vi "filter_logic_delays.vi"(9 "Filter Specific Constants":T2, 10 "Variables Cluster":T4, 11 "controls cluster":T1={"High Charge Limit"=0, "Low Charge Limit"=0, "Time Out Limit"=0, "High Velocity Count"=0, "Low Velocity Count"=0, "Sampling Rate"=26666666.59375, "High Mass Limit"=0, "Low Mass Limit"=0}) -> (3 "Output Cluster":T3)   [LabVIEW 2013]
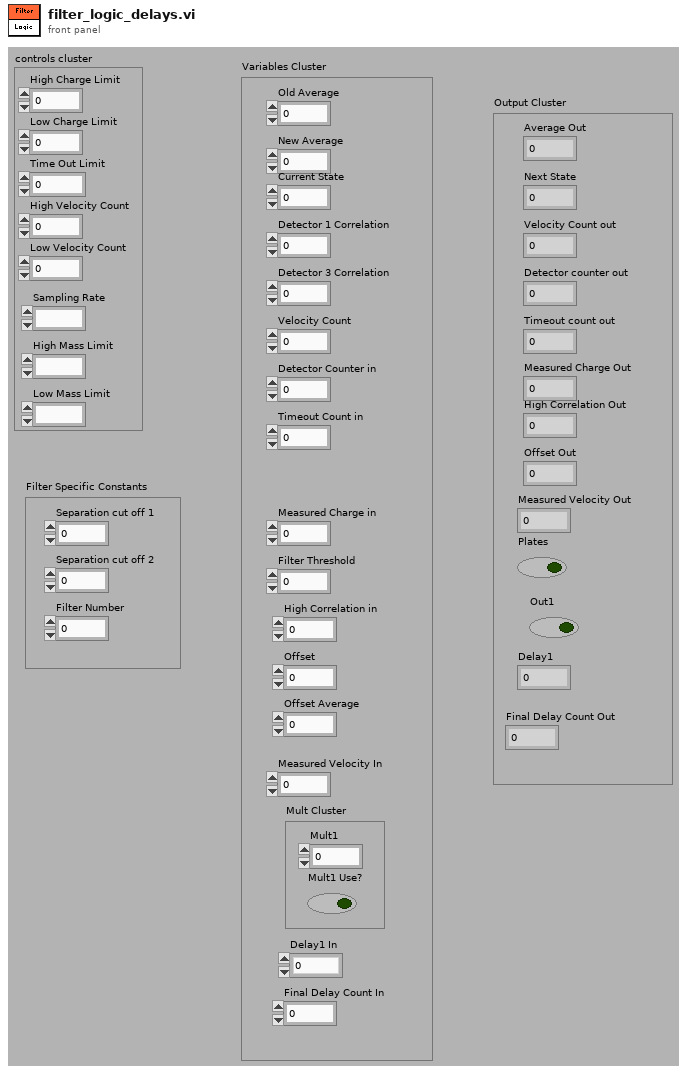
[diagram p1: front panel]
types:
  T1 = cluster{"High Charge Limit":i16, "Low Charge Limit":i16, "Time Out Limit":i32, "High Velocity Count":i32, "Low Velocity Count":i32, "Sampling Rate":fxp<+,30,25>, "High Mass Limit":i64, "Low Mass Limit":i64}
  T2 = cluster{"Separation cut off 1":i32, "Filter Number":i32, "Separation cut off 2":i32}
  T3 = cluster{"Average Out":i32, "Next State":u8, "Velocity Count out":i32, "Detector counter out":i32, "Timeout count out":u32, "Measured Charge Out":i32, "High Correlation Out":i32, "Plates":bool, "Offset Out":i32, "Measured Velocity Out":i32, "Final Delay Count Out":u16, "Out1":bool, "Delay1":i32}
  T4 = cluster{"Old Average":i32, "New Average":i32, "Current State":u8, "Detector 1 Correlation":i32, "Detector 3 Correlation":i32, "Velocity Count":i32, "Detector Counter in":i32, "Timeout Count in":i32, "Measured Charge in":i32, "Filter Threshold":i32, "High Correlation in":i32, "Offset":i32, "Offset Average":i32, "Measured Velocity In":i32, "Mult Cluster":cluster{"Mult1":fxp<+,16,7>, "Mult1 Use?":bool}, "Final Delay Count In":u16, "Delay1 In":i32}
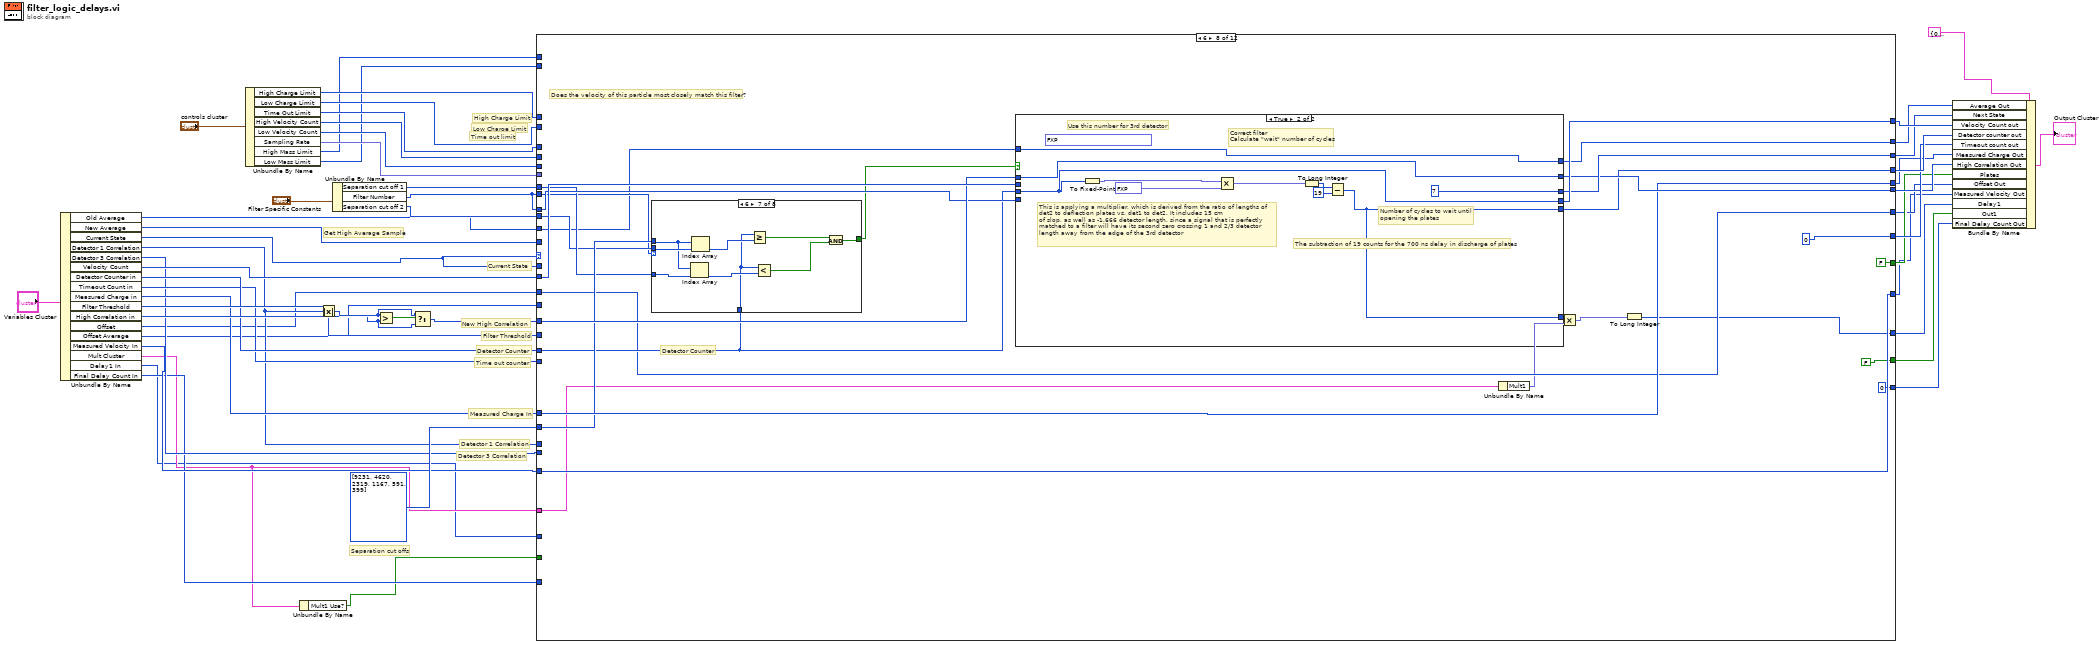
[diagram p0: block diagram]
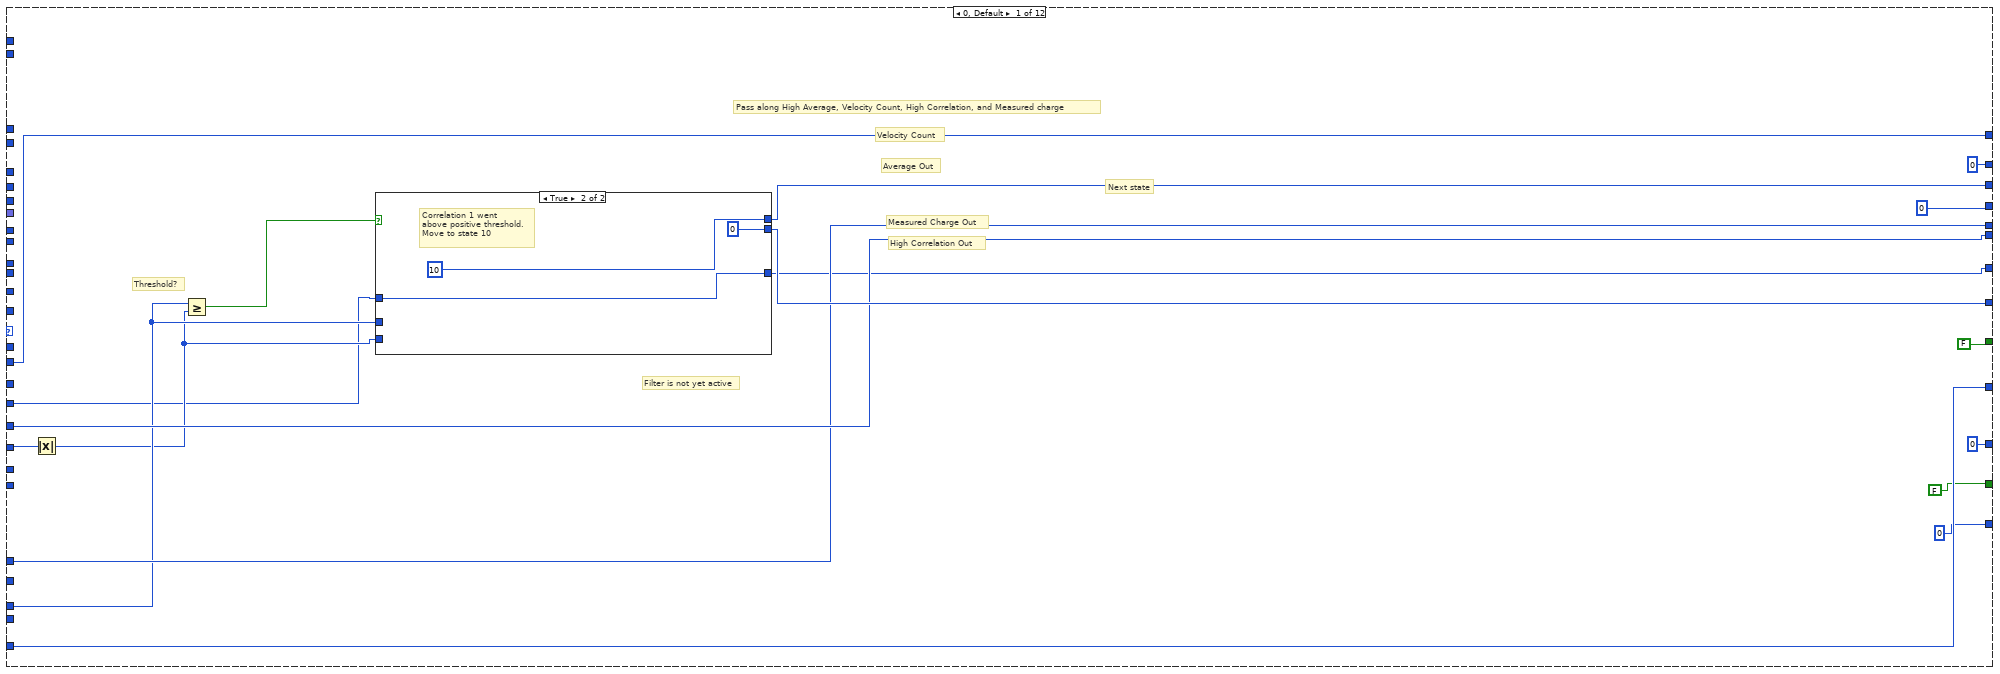
[diagram p2: hidden frame]
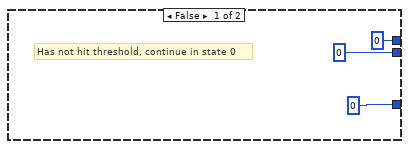
[diagram p3: hidden frame]
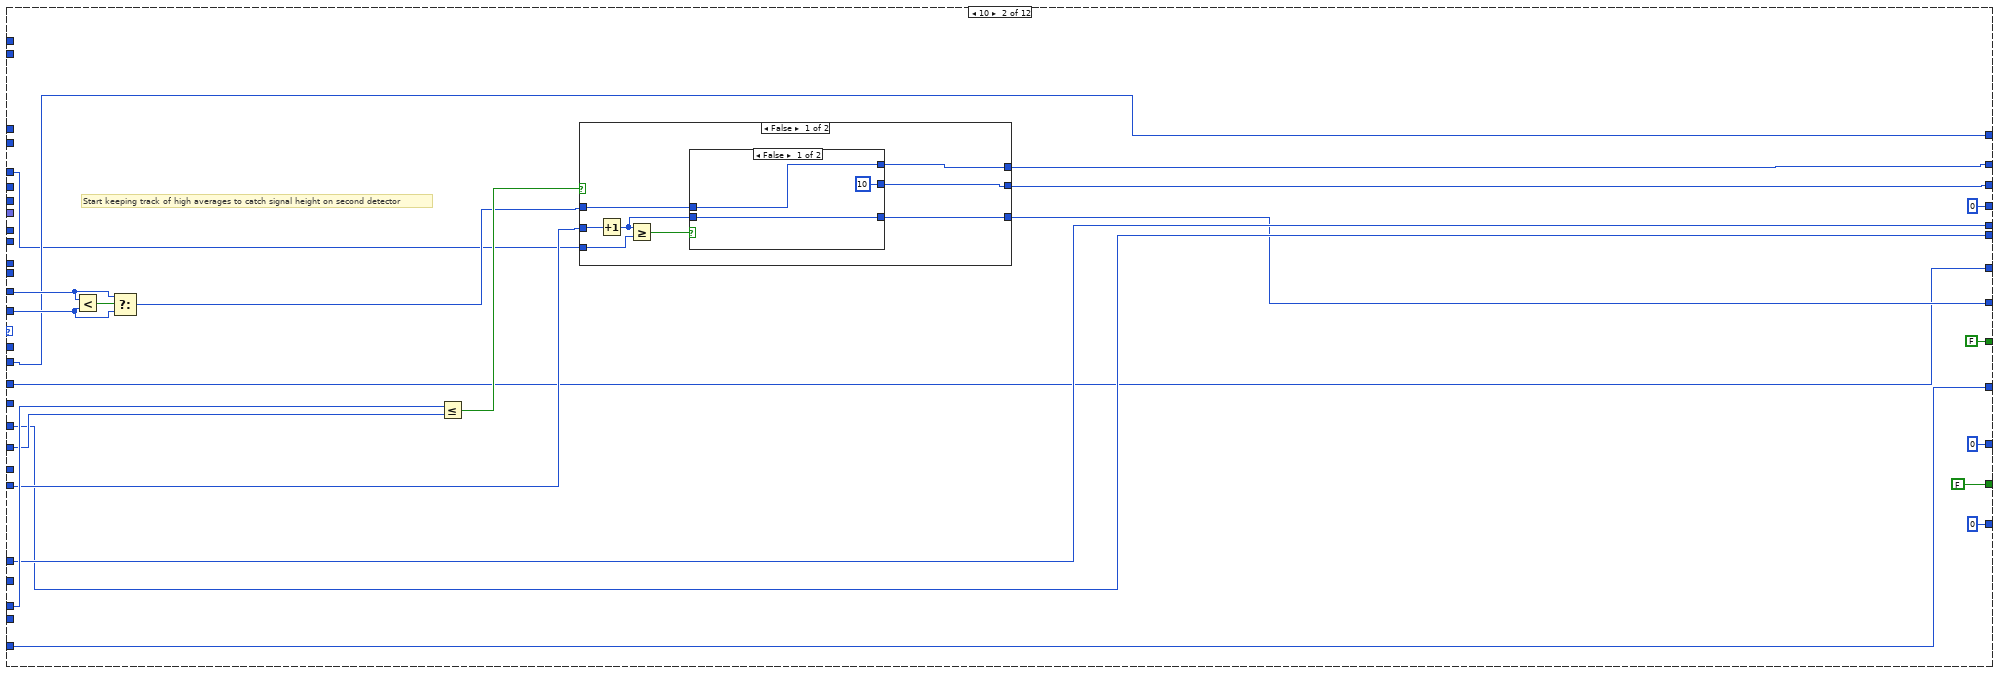
[diagram p4: hidden frame]
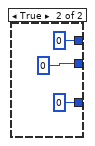
[diagram p5: hidden frame]
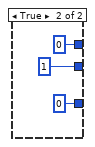
[diagram p6: hidden frame]
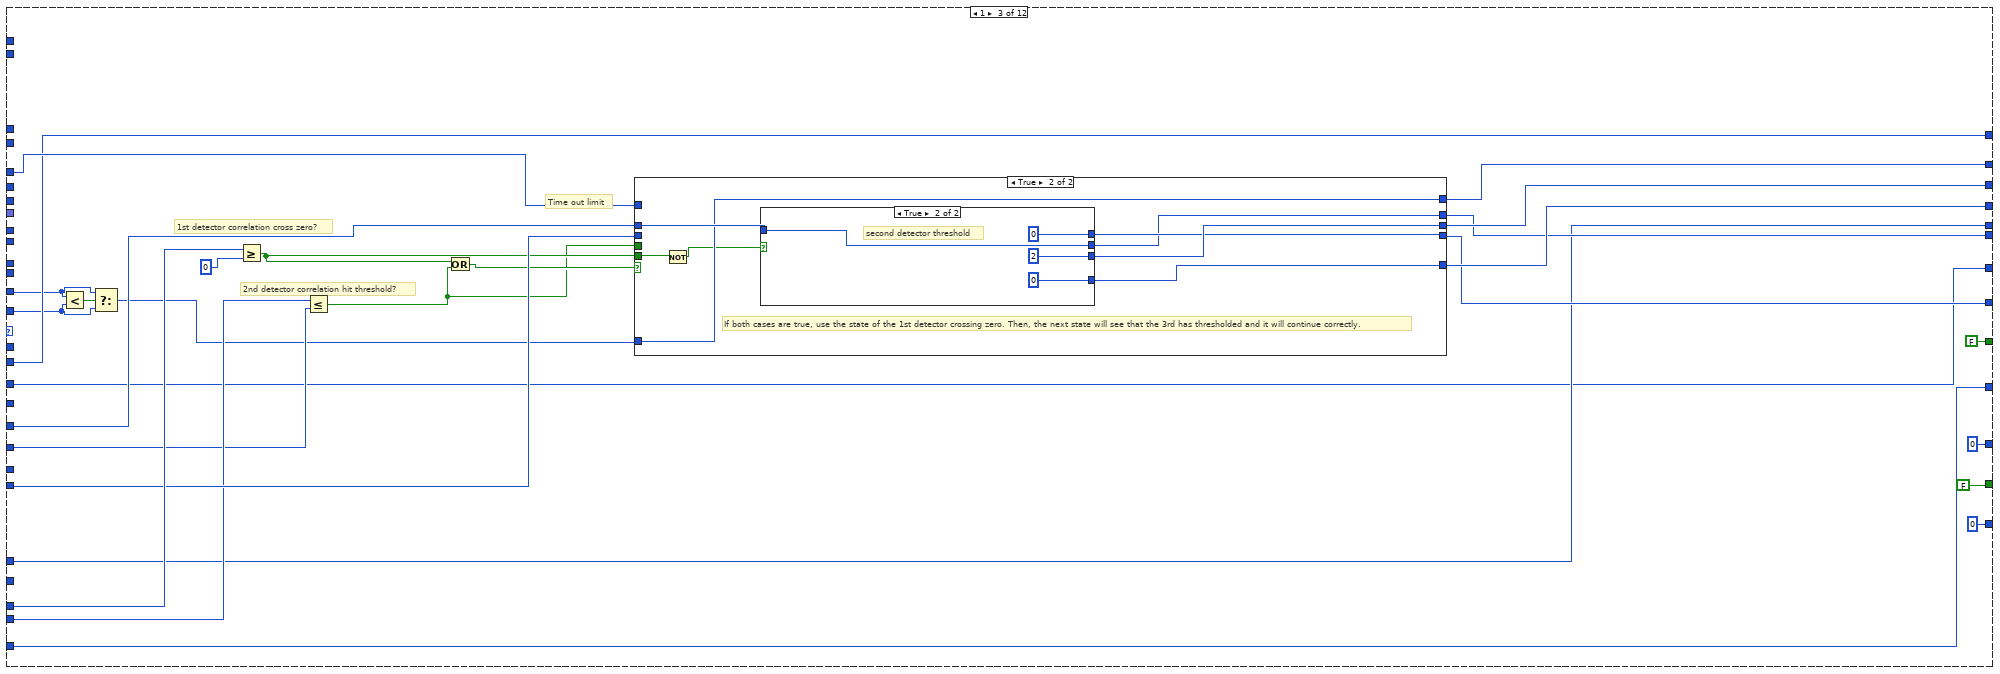
[diagram p7: hidden frame]
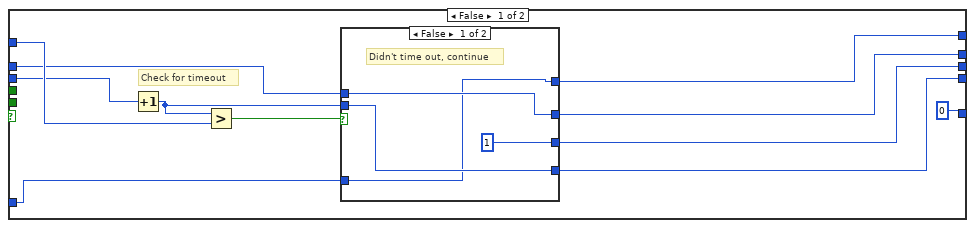
[diagram p8: hidden frame]
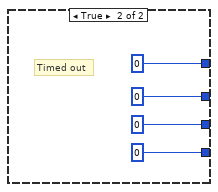
[diagram p9: hidden frame]
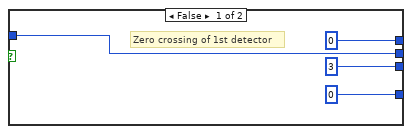
[diagram p10: hidden frame]
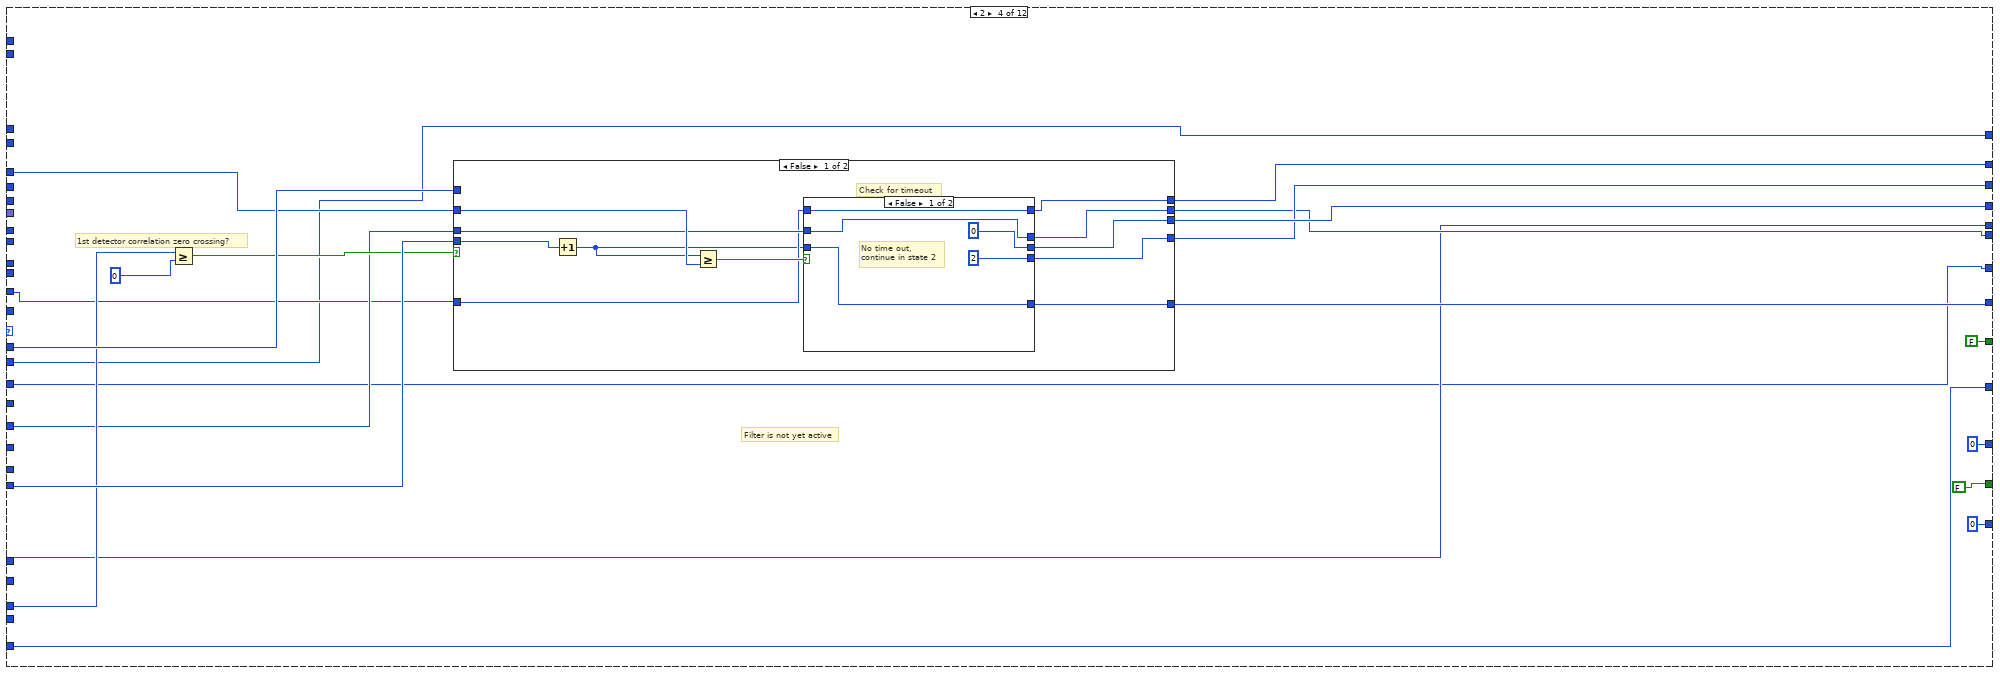
[diagram p11: hidden frame]
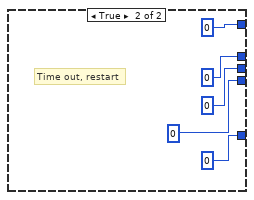
[diagram p12: hidden frame]
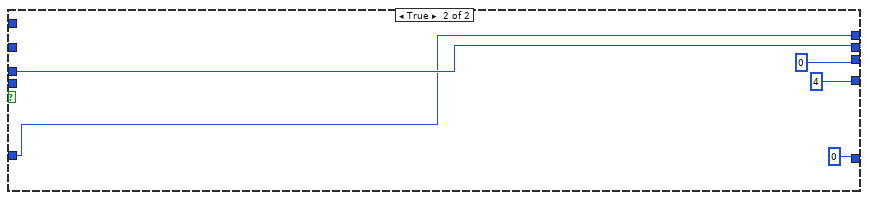
[diagram p13: hidden frame]
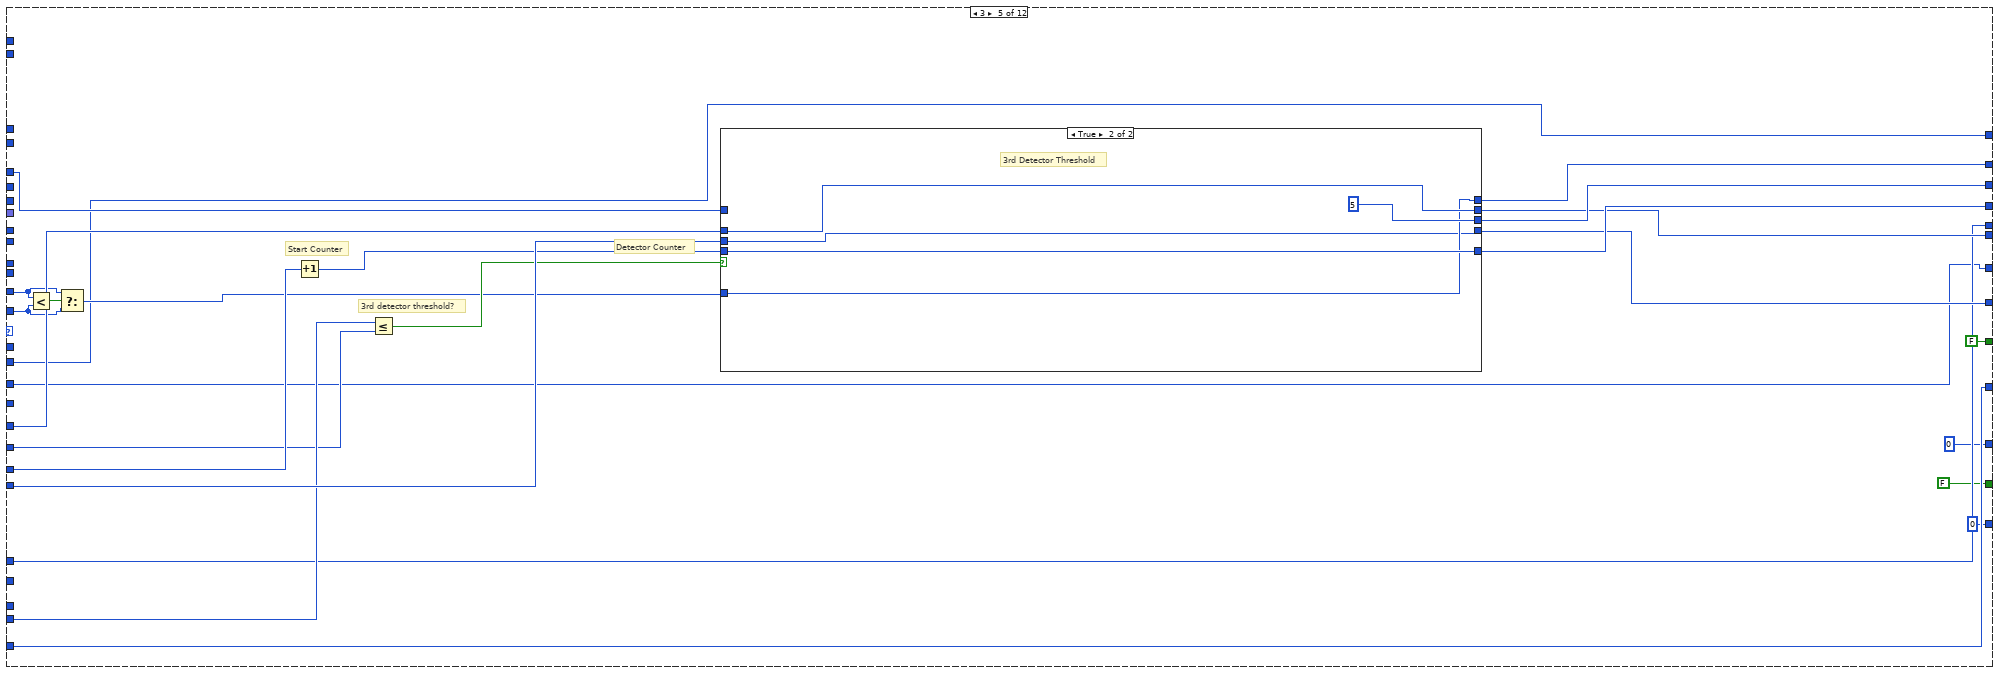
[diagram p14: hidden frame]
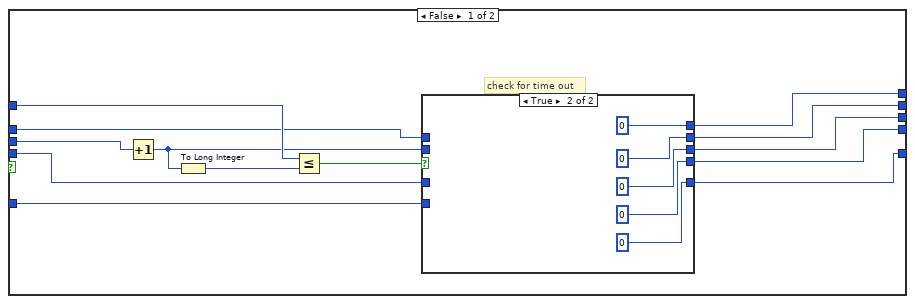
[diagram p15: hidden frame]
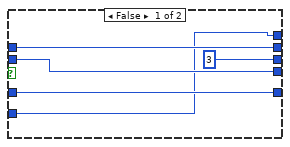
[diagram p16: hidden frame]
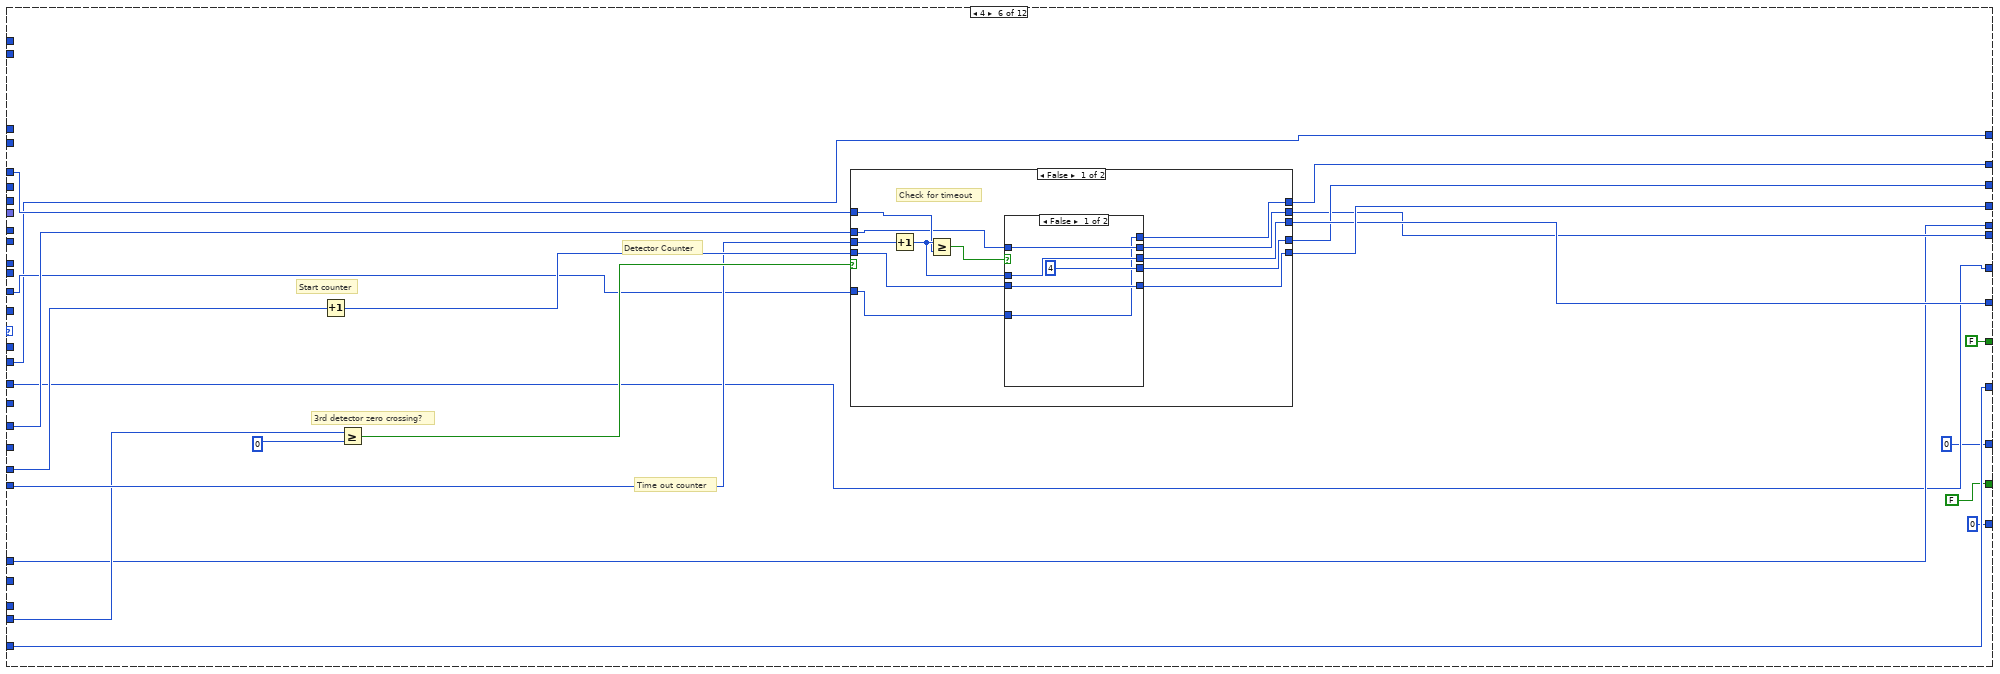
[diagram p17: hidden frame]
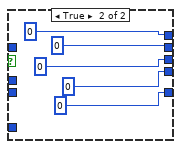
[diagram p18: hidden frame]
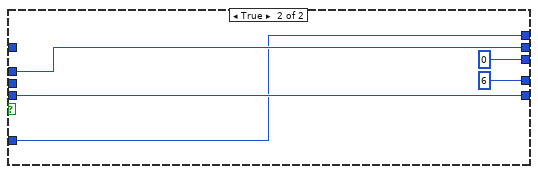
[diagram p19: hidden frame]
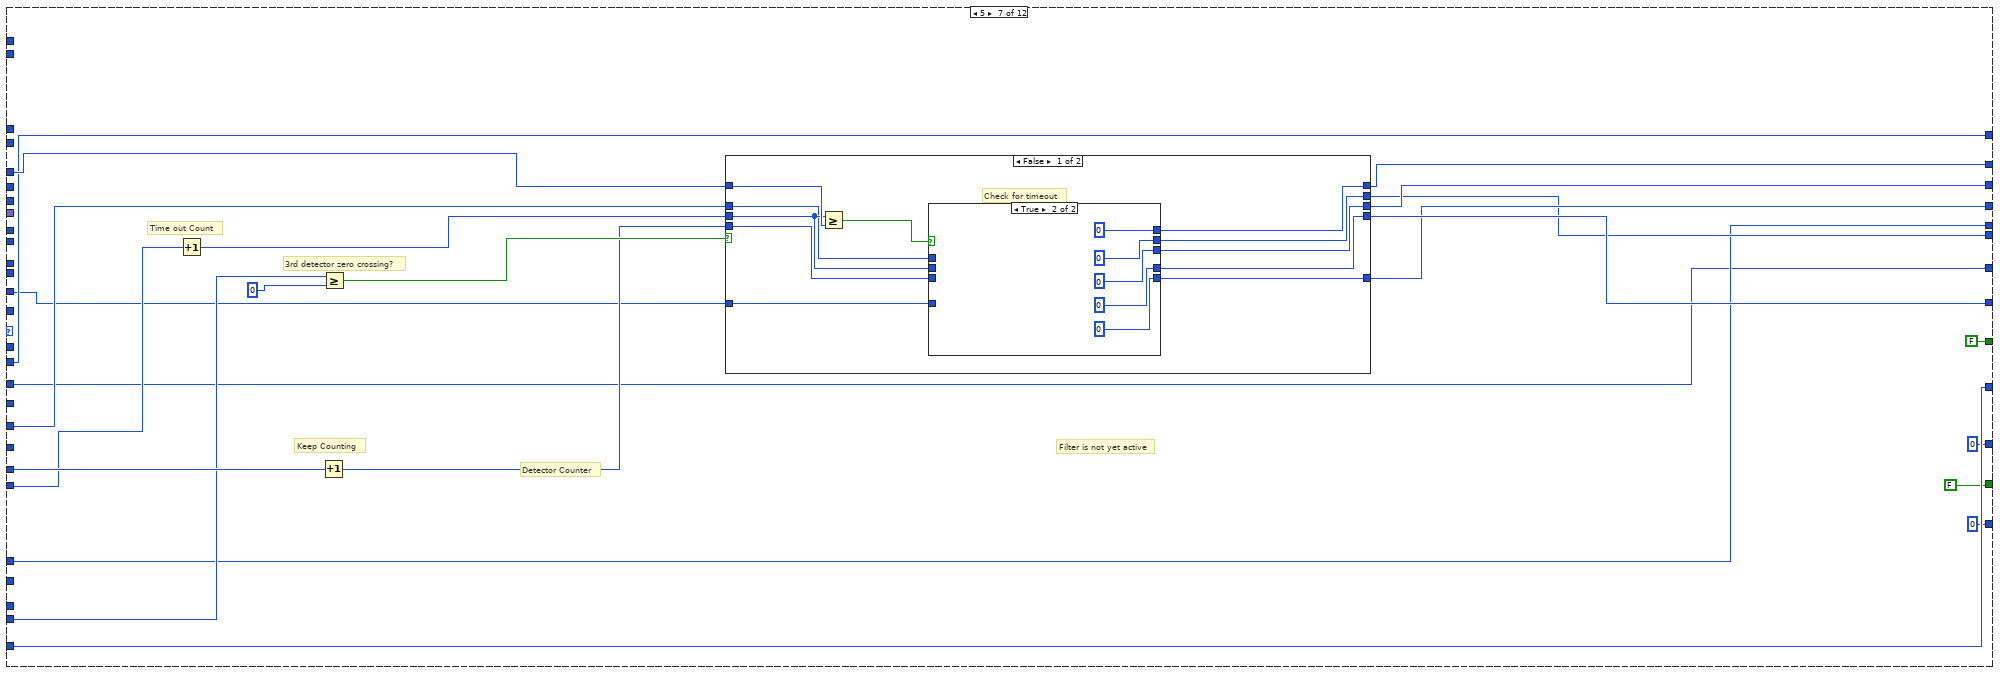
[diagram p20: hidden frame]
diagram:
  # "Detector 3 Correlation"
  # "Detector 1 Correlation"
  # "Separation cut offs"
  # "Measured Charge In"
  # "Time out counter"
  # "Detector Counter"
  # "Filter Threshold"
  # "New High Correlation"
  # "Current State"
  # "Get High Average Sample"
  # "Time out limit"
  # "Low Charge Limit"
  # "High Charge Limit"
  n1 = Unbundle By Name("Variables Cluster") -> ("Old Average"=w25:i32, "New Average"=w24:i32, "Current State"=w46:u8, "Detector 1 Correlation"=w35:i32, "Detector 3 Correlation"=w34:i32, "Velocity Count"=w45:i32, "Detector Counter in"=w39:i32, "Timeout Count in"=w38:i32, "Measured Charge in"=w37:i32, "Filter Threshold"=w40:i32, "High Correlation in"=w41:i32, "Offset"=w23:i32, "Offset Average"=w22:i32, "Measured Velocity In"=w19:i32, "Mult Cluster"=w7:cluster{"Mult1":fxp<+,16,7>, "Mult1 Use?":bool}, "Delay1 In"=w3:i32, "Final Delay Count In"=w8:u16)
  n2 = Unbundle By Name("controls cluster") -> ("High Charge Limit"=w18:i16, "Low Charge Limit"=w17:i16, "Time Out Limit"=w16:i32, "High Velocity Count"=w15:i32, "Low Velocity Count"=w14:i32, "Sampling Rate"=w13:fxp<+,30,25>, "High Mass Limit"=w12:i64, "Low Mass Limit"=w11:i64)
  n3 = Unbundle By Name(w7) -> ("Mult1 Use?"=w4:bool)
  n4 = Absolute Value(x=w35) -> (abs(x)=w42:i32)
  n5 = Unbundle By Name("Filter Specific Constants") -> ("Separation cut off 1"=w50:i32, "Filter Number"=w49:i32, "Separation cut off 2"=w48:i32)
  n6 = Greater?(x=w42, y=w41) -> (0:w43:bool)
  n7 = Select(t=w42, s=w43, f=w41) -> (s? t:f=w44:i32)
  n8 = case shown="6" w46 {
    tunnel: w35 -> [w61 w94 w141 w191 _ _ _ _ _ _ _ _]
    tunnel: w34 -> [_ _ w130 _ w240 w290 w338 _ _ _ _ _]
    tunnel: w40 -> [w59 w93 w129 _ w239 _ _ _ _ _ _ _]
    tunnel: w39 -> [_ _ _ _ w242 w298 w347 w389 w523 w566 w608 _]
    tunnel: [0 0 w139 w197 w248 w296 w340 w376 w522 w562 w604 0] -> w31
    tunnel: [w69 w91 w138 w196 w247 w293 w343 w398 w521 w564 w605 w645] -> w27
    tunnel: w46 -> [_ _ _ w195 _ _ _ _ _ _ _ _]
    tunnel: w45 -> [w65 w87 w131 w181 w228 w281 w339 w399 w486 w567 w602 w636]
    tunnel: w16 -> [_ w76 w137 w194 w245 w291 w344 _ _ _ _ _]
    tunnel: w38 -> [_ w90 w136 w193 w246 w292 w346 _ w510 _ _ _]
    tunnel: [w68 w82 w135 w192 w244 w294 w342 u32 0 w509 u32 0 ("Timeout Count in") u32 0 u32 0 ("Timeout Count in")] -> w30
    tunnel: w14 -> [_ _ _ _ _ _ _ _ w520 _ _ _]
    tunnel: w15 -> [_ _ _ _ _ _ _ _ w519 _ _ _]
    tunnel: [w65 w87 w131 w181 w228 w281 w339 w400 w518 w563 w602 w636] -> w33
    tunnel: i32[] [9231, 4620, 2319, 1167, 591, 399] -> [_ _ _ _ _ _ _ w392 _ _ _ _]
    tunnel: w17 -> [_ _ _ _ _ _ _ _ w517 _ _ _]
    tunnel: w18 -> [_ _ _ _ _ _ _ _ w516 _ _ _]
    tunnel: w44 -> [w64 w84 w128 w188 w238 w284 w336 w396 w515 w560 w600 _]
    tunnel: [w64 w84 w127 w187 w237 w288 w335 w397 w514 w560 w601 0 ("Noise Level")] -> w28
    tunnel: w37 -> [w63 w85 w126 w186 w236 w287 w334 w395 w513 w555 w596 w638]
    tunnel: [w63 w85 w126 w186 w236 w287 w334 w395 w512 w556 w596 w638] -> w29
    tunnel: [0 ("Old Average In") w88 w125 w185 w235 w286 w333 w394 w500 w552 0 ("Old Average In") 0 ("Old Average In")] -> w32
    tunnel: w50 -> [_ _ _ _ _ _ _ w391 _ _ _ _]
    tunnel: w49 -> [_ _ _ _ _ _ _ w393 _ _ _ _]
    tunnel: w49 -> [_ _ _ _ _ _ _ w387 w511 w565 w599 _]
    tunnel: w48 -> [_ _ _ _ _ _ _ w390 _ _ _ _]
    tunnel: [FALSE FALSE ("Data") FALSE FALSE FALSE FALSE FALSE FALSE w506 w559 w595 FALSE ("Data")] -> w26
    tunnel: w25 -> [_ w96 w122 w183 w232 w283 w331 w385 w500 w552 _ _]
    tunnel: w24 -> [_ w95 w121 _ w231 _ _ _ _ _ _ _]
    tunnel: w23 -> [_ w81 w119 w182 w229 w282 w330 w384 w501 w551 _ _]
    tunnel: w22 -> [w56 _ _ _ _ _ _ _ _ _ _ _]
    tunnel: [w57 w81 w119 w182 w229 w282 w330 w384 w501 w551 0 ("Offset") 0 ("Offset")] -> w21
    tunnel: [w55 w80 w118 w180 w227 w280 w329 w383 w503 w557 w593 w643] -> w20
    tunnel: w19 -> [w55 w80 w118 w180 w227 w280 w329 w383 w502 w558 w593 w643]
    tunnel: w13 -> [_ _ _ _ _ _ _ _ _ _ _ _]
    tunnel: w12 -> [_ _ _ _ _ _ _ _ w499 _ _ _]
    tunnel: w11 -> [_ _ _ _ _ _ _ _ w498 _ _ _]
    tunnel: w7 -> [_ _ _ _ _ _ _ w381 _ _ _ _]
    tunnel: w3 -> [_ _ _ _ _ _ _ _ w485 w550 w592 w634]
    tunnel: [0 0 0 0 0 0 0 w375 w484 w548 w591 w630] -> w5
    tunnel: [FALSE FALSE FALSE FALSE FALSE FALSE FALSE FALSE FALSE w544 w585 w635] -> w6
    tunnel: [u16 0 u16 0 u16 0 u16 0 u16 0 u16 0 u16 0 u16 0 u16 0 u16 0 w590 w644] -> w9
    tunnel: w8 -> [_ _ _ _ _ _ _ _ _ _ _ w631]
    tunnel: w4 -> [_ _ _ _ _ _ _ _ _ w545 w586 _]
    frame 0, Default {
      # "Filter is not yet active"
      # "High Correlation Out"
      # "Measured Charge Out"
      # "Next state"
      # "Average Out"
      # "Velocity Count"
      # "Pass along High Average, Velocity Count, High Correlation, and Measured charge"
      # "Threshold?"
      n9 = Absolute Value(x=w59) -> (abs(x)=w58:i32)
      n10 = Greater Or Equal?(x=w61, y=w58) -> (x >= y?=w66:bool)
      n11 = case shown="True" w66 {
        tunnel: [u8 0 u8 10] -> w69
        tunnel: [u32 0 u32 0] -> w68
        tunnel: w61 -> [_ _]
        tunnel: w58 -> [_ _]
        tunnel: [0 w73] -> w57
        tunnel: w56 -> [_ w73]
        frame False {
          # "Has not hit threshold, continue in state 0"
        }
        frame True {
          # "Correlation 1 went\nabove positive threshold.\nMove to state 10"
        }
      }
    }
    frame 10 {
      # "Start keeping track of high averages to catch signal height on second detector"
      n12 = Less?(x=w96, y=w95) -> (x < y?=w97:bool)
      n13 = Select(t=w96, s=w97, f=w95) -> (s? t:f=w89:i32)
      n14 = Less Or Equal?(x=w94, y=w93) -> (x <= y?=w92:bool)
      n15 = case shown="False" w92 {
        tunnel: [w103 u8 1] -> w91
        tunnel: w90 -> [w100 _]
        tunnel: w76 -> [w105 _]
        tunnel: w89 -> [w102 _]
        tunnel: [w101 0 ("New Average")] -> w88
        tunnel: [w98 0] -> w82
        frame False {
          n16 = Increment(x=w100) -> (x+1=w99:i32)
          n17 = Greater Or Equal?(x=w99, y=w105) -> (x >= y?=w104:bool)
          n18 = case shown="False" w104 {
            tunnel: [u8 10 u8 0] -> w103
            tunnel: w102 -> [w108 _]
            tunnel: [w108 0 ("New Average")] -> w101
            tunnel: w99 -> [w106 _]
            tunnel: [w106 0] -> w98
            frame False {
            }
            frame True {
            }
          }
        }
        frame True {
        }
      }
    }
    frame 1 {
      # "Time out limit"
      # "2nd detector correlation hit threshold?"
      # "1st detector correlation cross zero?"
      n19 = Less?(x=w122, y=w121) -> (x < y?=w123:bool)
      n20 = Select(t=w122, s=w123, f=w121) -> (s? t:f=w120:i32)
      n21 = Greater Or Equal?(x=w141, y=0) -> (x >= y?=w133:bool)
      n22 = Less Or Equal?(x=w130, y=w129) -> (x <= y?=w132:bool)
      n23 = Or(x=w133, y=w132) -> (x .or. y?=w134:bool)
      n24 = case shown="True" w134 {
        tunnel: [0 w167] -> w139
        tunnel: [w150 w168] -> w138
        tunnel: w137 -> [w152 _]
        tunnel: w136 -> [w149 _]
        tunnel: [w148 w166] -> w135
        tunnel: w133 -> [_ w162]
        tunnel: w132 -> [_ _]
        tunnel: w128 -> [w146 w165]
        tunnel: [w145 w164] -> w127
        tunnel: [w144 w163] -> w125
        tunnel: w120 -> [w142 w163]
        frame False {
          # "Check for timeout"
          n25 = Increment(x=w149) -> (x+1=w143:i32)
          n26 = Greater?(x=w143, y=w152) -> (0:w151:bool)
          n27 = case shown="False" w151 {
            tunnel: [u8 1 u8 0] -> w150
            tunnel: w143 -> [w155 _]
            tunnel: [w155 u32 0] -> w148
            tunnel: w146 -> [w154 _]
            tunnel: [w154 0 ("High Correlation In")] -> w145
            tunnel: [w153 0 ("Old Average In")] -> w144
            tunnel: w142 -> [w153 _]
            frame False {
              # "Didn't time out, continue"
            }
            frame True {
              # "Timed out"
            }
          }
        }
        frame True {
          # "If both cases are true, use the state of the 1st detector crossing zero. Then, the next state will see that the 3rd has thresholded and it will continue correctly."
          n28 = Not(x=w162) -> (.not. x?=w161:bool)
          n29 = case shown="True" w161 {
            tunnel: [u8 3 u8 2] -> w168
            tunnel: [0 0] -> w167
            tunnel: [u32 0 u32 0] -> w166
            tunnel: w165 -> [w169 w173]
            tunnel: [w169 w173] -> w164
            frame False {
              # "Zero crossing of 1st detector"
            }
            frame True {
              # "second detector threshold"
            }
          }
        }
      }
    }
    frame 2 {
      # "Filter is not yet active"
      # "1st detector correlation zero crossing?"
      n30 = Greater Or Equal?(x=w191, y=0) -> (x >= y?=w189:bool)
      n31 = case shown="False" w189 {
        tunnel: [w203 0] -> w197
        tunnel: [w207 u8 4] -> w196
        tunnel: w195 -> [_ _]
        tunnel: w194 -> [w206 _]
        tunnel: w193 -> [w204 _]
        tunnel: [w205 u32 0] -> w192
        tunnel: w188 -> [w202 w220]
        tunnel: [w201 w220] -> w187
        tunnel: [w200 w219] -> w185
        tunnel: w183 -> [w199 w219]
        frame False {
          # "Check for timeout"
          n32 = Increment(x=w204) -> (x+1=w198:i32)
          n33 = Greater Or Equal?(x=w198, y=w206) -> (x >= y?=w208:bool)
          n34 = case shown="False" w208 {
            tunnel: [u8 2 u8 0] -> w207
            tunnel: w198 -> [w213 _]
            tunnel: [w213 u32 0] -> w205
            tunnel: [0 0] -> w203
            tunnel: w202 -> [w210 _]
            tunnel: [w210 0 ("High Correlation In")] -> w201
            tunnel: [w209 0 ("Old Average In")] -> w200
            tunnel: w199 -> [w209 _]
            frame False {
              # "No time out, \ncontinue in state 2"
            }
            frame True {
              # "Time out, restart"
            }
          }
        }
        frame True {
        }
      }
    }
    frame 3 {
      # "3rd detector threshold?"
      # "Start Counter"
      # "Detector Counter"
      n35 = Less?(x=w232, y=w231) -> (x < y?=w233:bool)
      n36 = Select(t=w232, s=w233, f=w231) -> (s? t:f=w230:i32)
      n37 = Increment(x=w242) -> (x+1=w241:i32)
      n38 = Less Or Equal?(x=w240, y=w239) -> (x <= y?=w243:bool)
      n39 = case shown="True" w243 {
        tunnel: w241 -> [w256 w276]
        tunnel: [w255 w276] -> w248
        tunnel: [w258 u8 5] -> w247
        tunnel: w246 -> [w254 w272]
        tunnel: w245 -> [w261 _]
        tunnel: [w257 w272] -> w244
        tunnel: w238 -> [w252 w274]
        tunnel: [w251 w274] -> w237
        tunnel: [w250 w273] -> w235
        tunnel: w230 -> [w249 w273]
        frame False {
          # "check for time out"
          n40 = Increment(x=w254) -> (x+1=w253:i32)
          n41 = To Long Integer(number=w253) -> (32bit integer=w260:i32)
          n42 = Less Or Equal?(x=w261, y=w260) -> (x <= y?=w259:bool)
          n43 = case shown="True" w259 {
            tunnel: [u8 3 u8 0] -> w258
            tunnel: w253 -> [w265 _]
            tunnel: [w265 u32 0] -> w257
            tunnel: w256 -> [w264 _]
            tunnel: [w264 0] -> w255
            tunnel: w252 -> [w263 _]
            tunnel: [w263 0 ("High Correlation In")] -> w251
            tunnel: [w262 0 ("Old Average In")] -> w250
            tunnel: w249 -> [w262 _]
            frame False {
            }
            frame True {
            }
          }
        }
        frame True {
          # "3rd Detector Threshold"
        }
      }
    }
    frame 4 {
      # "Time out counter"
      # "3rd detector zero crossing?"
      # "Start counter"
      # "Detector Counter"
      n44 = Increment(x=w298) -> (x+1=w295:i32)
      n45 = Greater Or Equal?(x=w290, y=0) -> (x >= y?=w297:bool)
      n46 = case shown="False" w297 {
        tunnel: [w303 w325] -> w296
        tunnel: w295 -> [w304 w325]
        tunnel: [w306 u32 0] -> w294
        tunnel: [w308 u8 6] -> w293
        tunnel: w292 -> [w310 _]
        tunnel: w291 -> [w305 _]
        tunnel: w284 -> [w302 w322]
        tunnel: [w301 w322] -> w288
        tunnel: [w300 w321] -> w286
        tunnel: w283 -> [w299 w321]
        frame False {
          # "Check for timeout"
          n47 = Increment(x=w310) -> (x+1=w307:i32)
          n48 = Greater Or Equal?(x=w307, y=w305) -> (x >= y?=w309:bool)
          n49 = case shown="False" w309 {
            tunnel: [u8 4 u8 0] -> w308
            tunnel: w307 -> [w314 _]
            tunnel: [w314 u32 0] -> w306
            tunnel: w304 -> [w313 _]
            tunnel: [w313 0] -> w303
            tunnel: w302 -> [w312 _]
            tunnel: [w312 0 ("High Correlation In")] -> w301
            tunnel: [w311 0 ("Old Average In")] -> w300
            tunnel: w299 -> [w311 _]
            frame False {
            }
            frame True {
            }
          }
        }
        frame True {
        }
      }
    }
    frame 5 {
      # "Filter is not yet active"
      # "Time out Count"
      # "3rd detector zero crossing?"
      # "Keep Counting"
      # "Detector Counter"
      n50 = Increment(x=w346) -> (x+1=w345:i32)
      n51 = Increment(x=w347) -> (x+1=w341:i32)
      n52 = Greater Or Equal?(x=w338, y=0) -> (x >= y?=w348:bool)
      n53 = case shown="False" w348 {
        tunnel: w345 -> [w355 _]
        tunnel: w344 -> [w359 _]
        tunnel: [w357 u8 6] -> w343
        tunnel: [w356 u32 0] -> w342
        tunnel: w341 -> [w354 w372]
        tunnel: [w353 w372] -> w340
        tunnel: w336 -> [w351 w371]
        tunnel: [w352 w371] -> w335
        tunnel: [w350 w370] -> w333
        tunnel: w331 -> [w349 w370]
        frame False {
          # "Check for timeout"
          n54 = Greater Or Equal?(x=w355, y=w359) -> (x >= y?=w358:bool)
          n55 = case shown="True" w358 {
            tunnel: [u8 5 u8 0] -> w357
            tunnel: [w363 u32 0] -> w356
            tunnel: w355 -> [w363 _]
            tunnel: w354 -> [w362 _]
            tunnel: [w362 0] -> w353
            tunnel: [w361 0 ("High Correlation In")] -> w352
            tunnel: w351 -> [w361 _]
            tunnel: [w360 0 ("Old Average In")] -> w350
            tunnel: w349 -> [w360 _]
            frame False {
            }
            frame True {
            }
          }
        }
        frame True {
        }
      }
    }
    frame 6 {
      # "Does the velocity of this particle most closely match this filter?"
      # "Detector Counter"
      n56 = case shown="6" w387 {
        tunnel: w392 -> [w409 w415 w419 w428 w438 w446 w455 w465]
        tunnel: w391 -> [w408 w414 w418 w427 w436 w445 w454 w464]
        tunnel: w390 -> [w407 _ w420 w429 w437 w447 w456 _]
        tunnel: w389 -> [w405 w413 w417 w426 w435 w444 w453 w462]
        tunnel: [w404 w411 w416 w425 w434 w443 w452 w461] -> w388
        frame 0, Default {
          n57 = Index Array(array=w409, index=w408) -> (element=w406:i32)
          n58 = Index Array(array=w409, index=w407) -> (element=w410:i32)
          n59 = Greater Or Equal?(x=w405, y=w410) -> (x >= y?=w403:bool)
          n60 = Less?(x=w405, y=w406) -> (x < y?=w402:bool)
          n61 = And(x=w403, y=w402) -> (x .and. y?=w404:bool)
        }
        frame 1 {
          n62 = Index Array(array=w415, index=w414) -> (element=w412:i32)
          n63 = Greater Or Equal?(x=w413, y=w412) -> (x >= y?=w411:bool)
        }
        frame 2 {
          n64 = Index Array(array=w419, index=w418) -> (element=w422:i32)
          n65 = Index Array(array=w419, index=w420) -> (element=w421:i32)
          n66 = Greater Or Equal?(x=w417, y=w421) -> (x >= y?=w423:bool)
          n67 = Less?(x=w417, y=w422) -> (x < y?=w424:bool)
          n68 = And(x=w423, y=w424) -> (x .and. y?=w416:bool)
        }
        frame 3 {
          n69 = Index Array(array=w428, index=w427) -> (element=w431:i32)
          n70 = Index Array(array=w428, index=w429) -> (element=w430:i32)
          n71 = Greater Or Equal?(x=w426, y=w430) -> (x >= y?=w432:bool)
          n72 = Less?(x=w426, y=w431) -> (x < y?=w433:bool)
          n73 = And(x=w432, y=w433) -> (x .and. y?=w425:bool)
        }
        frame 4 {
          # "3"
          # "2"
          n74 = Index Array(array=w438, index=w436) -> (element=w440:i32)
          n75 = Index Array(array=w438, index=w437) -> (element=w439:i32)
          n76 = Greater Or Equal?(x=w435, y=w439) -> (x >= y?=w441:bool)
          n77 = Less?(x=w435, y=w440) -> (x < y?=w442:bool)
          n78 = And(x=w441, y=w442) -> (x .and. y?=w434:bool)
        }
        frame 5 {
          n79 = Index Array(array=w446, index=w445) -> (element=w449:i32)
          n80 = Index Array(array=w446, index=w447) -> (element=w448:i32)
          n81 = Greater Or Equal?(x=w444, y=w448) -> (x >= y?=w450:bool)
          n82 = Less?(x=w444, y=w449) -> (x < y?=w451:bool)
          n83 = And(x=w450, y=w451) -> (x .and. y?=w443:bool)
        }
        frame 6 {
          n84 = Index Array(array=w455, index=w454) -> (element=w459:i32)
          n85 = Index Array(array=w455, index=w456) -> (element=w460:i32)
          n86 = Greater Or Equal?(x=w453, y=w460) -> (x >= y?=w458:bool)
          n87 = Less?(x=w453, y=w459) -> (x < y?=w457:bool)
          n88 = And(x=w458, y=w457) -> (x .and. y?=w452:bool)
        }
        frame 7 {
          n89 = Index Array(array=w465, index=w464) -> (element=w463:i32)
          n90 = Less?(x=w462, y=w463) -> (x < y?=w461:bool)
        }
      }
      n91 = case shown="True" w388 {
        tunnel: [0 w472] -> w376
        tunnel: w389 -> [_ w479]
        tunnel: [w471 w479] -> w400
        tunnel: w399 -> [w471 _]
        tunnel: [u8 0 u8 7] -> w398
        tunnel: [0 ("High Correlation In") w477] -> w397
        tunnel: w396 -> [_ w477]
        tunnel: [0 ("Old Average In") w476] -> w394
        tunnel: w393 -> [_ _]
        tunnel: w385 -> [_ w476]
        tunnel: [0 w472] -> w377
        frame False {
          # "Incorrect filter, restart"
        }
        frame True {
          (unwired) fxp<+,31,3> 7.340293329209089
          # "The subtraction of 19 counts for the 700 ns delay in discharge of plates"
          # "Use this number for 3rd detector"
          # "Number of cycles to wait until\nopening the plates"
          # "This is applying a multiplier, which is derived from the ratio of lengths of\ndet2 to deflection plates vs. det1 to det2. It includes 15 cm\nof slop, as well as -1.666 detector length, since a signal that is perfectly\nmatched to a filter will have its second zero crossing 1 and 2/3 detector \nlength away from the edge of the 3rd detector"
          # "Correct filter\nCalculate \"wait\" number of cycles"
          n92 = To Fixed-Point(number=w479) -> (fixed-point=w481:fxp<+/-,32,32>)  [unwired: 1 in]
          n93 = Multiply(x=w481, y=fxp<+,6,1> 1.40625) -> (x*y=w480:fxp<+/-,38,33>)
          n94 = To Long Integer(number=w480) -> (32bit integer=w474:i32)
          n95 = Subtract(x=w474, y=19) -> (x-y=w472:i32)
        }
      }
      n96 = Unbundle By Name(w381) -> ("Mult1"=w379:fxp<+,16,7>)
      n97 = Multiply(x=w377, y=w379) -> (x*y=w380:fxp<+/-,48,39>)
      n98 = To Long Integer(number=w380) -> (32bit integer=w375:i32)
    }
    frame 7 {
      # "Did the particle meet the mass conditions?"
      # "calculated mass of particle"
      # "Get charge from smoothed data"
      # "Check Velocity Conditions"
      # "Check Charge Conditions"
      # "Detector Counter"
      n99 = Subtract(x=w501, y=w500) -> (x-y=w505:i32)
      n100 = Square(x=w486) -> (x^2=w490:i32)
      n101 = To Quad Integer(1:w490) -> (0:w489:i64)
      n102 = Absolute Value(x=w505) -> (abs(x)=w487:i32)
      n103 = To Quad Integer(1:w487) -> (0:w488:i64)
      n104 = Multiply(x=w489, y=w488) -> (x*y=w491:i64)
      n105 = Less Or Equal?(x=w491, y=w499) -> (x <= y?=w492:bool)
      n106 = Greater Or Equal?(x=w491, y=w498) -> (x >= y?=w493:bool)
      n107 = Greater Or Equal?(x=w486, y=w519) -> (x >= y?=w494:bool)
      n108 = Less Or Equal?(x=w486, y=w520) -> (x <= y?=w495:bool)
      n109 = To Word Integer(number=w487) -> (16bit integer=w508:i16)
      n110 = To Word Integer(number=w487) -> (16bit integer=w507:i16)
      n111 = Less Or Equal?(x=w517, y=w508) -> (x <= y?=w496:bool)
      n112 = Greater Or Equal?(x=w516, y=w507) -> (x >= y?=w497:bool)
      n113 = Compound Arithmetic op=AND(w492, w493, w494, w495, w496, w497) -> (w504:bool)
      n114 = case shown="True" w504 {
        tunnel: w523 -> [_ w543]
        tunnel: w486 -> [w531 w537]
        tunnel: [0 w541] -> w522
        tunnel: [u8 0 u8 8] -> w521
        tunnel: [w531 w537] -> w518
        tunnel: w515 -> [_ w542]
        tunnel: [0 ("High Correlation In") w542] -> w514
        tunnel: w513 -> [w528 w535]
        tunnel: w487 -> [_ _]
        tunnel: [w528 w535] -> w512
        tunnel: w511 -> [_ _]
        tunnel: w510 -> [_ _]
        tunnel: [u32 0 ("Timeout Count in") 0 ("Timeout Count in")] -> w509
        tunnel: [FALSE ("Data") FALSE ("Data")] -> w506
        tunnel: [w525 w536] -> w503
        tunnel: w502 -> [w525 w536]
        tunnel: w485 -> [_ w534]
        tunnel: [0 w533] -> w484
        frame False {
          # "Correct filter, but wrong velocity and/or charge."
          # "Did not meet conditions, restart"
        }
        frame True {
          # "Met Conditions"
          # "Count \"Detector Counter\" down"
          n115 = Decrement(x=w534) -> (x-1=w533:i32)
          n116 = Decrement(x=w543) -> (x-1=w541:i32)
        }
      }
    }
    frame 8 {
      # "Met Conditions, count down until opening the plates"
      # "Count \"Detector Counter\" down"
      # "velocity count"
      n117 = Decrement(x=w550) -> (x-1=w548:i32)
      n118 = Subtract(x=w551, y=w552) -> (x-y=w554:i32)
      n119 = Absolute Value(x=w554) -> (abs(x)=w553:i32)
      n120 = Less Or Equal?(x=w548, y=0) -> (x <= y?=w546:bool)
      n121 = And(x=w545, y=w546) -> (x .and. y?=w544:bool)
      n122 = Decrement(x=w566) -> (x-1=w568:i32)
      n123 = Less Or Equal?(x=w568, y=0) -> (x <= y?=w569:bool)
      n124 = case shown="True" w569 {
        tunnel: [u8 8 u8 9] -> w564
        tunnel: [w576 w583] -> w562
        tunnel: w567 -> [w574 w578]
        tunnel: w568 -> [w576 _]
        tunnel: [w574 w578] -> w563
        tunnel: w565 -> [_ _]
        tunnel: [FALSE ("Data") TRUE ("Data")] -> w559
        tunnel: w558 -> [w572 _]
        tunnel: [w572 w578] -> w557
        tunnel: [w571 w577] -> w556
        tunnel: w555 -> [w571 _]
        tunnel: w553 -> [_ w577]
        frame False {
          # "Counting down to wait to open the plates"
        }
        frame True {
          # "velocity count"
          # "Number derived from ratio of lengths of plates (w/ 25cm of slop)\n vs. det1 to det3"
          # "clock counts to wait \nuntil close."
          n125 = To Fixed-Point(number=w578) -> (fixed-point=w580:fxp<+/-,32,32>)  [unwired: 1 in]
          n126 = Multiply(x=w580, y=fxp<+,2,1> 1.5 ("x")) -> (x*y=w584:fxp<+/-,34,33>)
          n127 = To Long Integer(number=w584) -> (32bit integer=w583:i32)
        }
      }
    }
    frame 9 {
      # "Count down and then close plates"
      # "Detector Counter"
      n128 = Decrement(x=w592) -> (x-1=w589:i32)
      n129 = Less Or Equal?(x=w589, y=0) -> (x <= y?=w587:bool)
      n130 = Decrement(x=w608) -> (x-1=w603:i32)
      n131 = And(x=w586, y=w587) -> (x .and. y?=w585:bool)
      n132 = Less Or Equal?(x=w603, y=0) -> (x <= y?=w606:bool)
      n133 = case shown="True" w606 {
        tunnel: [w613 0] -> w604
        tunnel: [u8 9 w618] -> w605
        tunnel: w603 -> [w613 _]
        tunnel: w600 -> [w612 _]
        tunnel: [w612 0 ("Noise Level")] -> w601
        tunnel: w599 -> [_ _]
        tunnel: [TRUE ("Data") FALSE ("Data")] -> w595
        tunnel: w589 -> [w610 w617]
        tunnel: w586 -> [_ w619]
        tunnel: [w610 w616] -> w591
        tunnel: [u16 0 w615] -> w590
        frame False {
          # "Count down to wait to close the plates"
        }
        frame True {
          # "Close plates here"
          n134 = case shown="True" w619 {
            tunnel: [u8 0 u8 12] -> w618
            tunnel: w617 -> [_ w627]
            tunnel: [0 w627] -> w616
            tunnel: [u16 0 u16 550] -> w615
            frame False {
            }
            frame True {
              # "Go to Delay State"
            }
          }
        }
      }
    }
    frame 12 {
      n135 = Decrement(x=w634) -> (x-1=w629:i32)
      n136 = Less Or Equal?(x=w629, y=0) -> (x <= y?=w632:bool)
      n137 = case shown="False" w632 {
        tunnel: [FALSE w655] -> w635
        tunnel: [u8 12 w654] -> w645
        tunnel: w631 -> [w649 w658]
        tunnel: [w649 w653] -> w644
        tunnel: [w647 0] -> w630
        tunnel: w629 -> [w647 _]
        frame False {
        }
        frame True {
          n138 = Decrement(x=w658) -> (x-1=w652:u16)
          n139 = Less Or Equal?(x=w652, y=u16 0) -> (x <= y?=w656:bool)
          n140 = case shown="False" w656 {
            tunnel: [TRUE FALSE] -> w655
            tunnel: [u8 12 u8 0] -> w654
            tunnel: [w659 u16 0] -> w653
            tunnel: w652 -> [w659 _]
            frame False {
            }
            frame True {
            }
          }
        }
      }
    }
  }
  n141 = Bundle By Name(cluster=T3 {"Average Out"=0, "Next State"=0, "Velocity Count out"=0, "Detector counter out"=0, "Timeout count out"=0, "Measured Charge Out"=0, "High Correlation Out"=0, "Plates"=FALSE, "Offset Out"=0, "Measured Velocity Out"=0, "Final Delay Count Out"=0, "Out1"=FALSE, "Delay1"=0} ("Output Cluster"), "Average Out"=w32, "Next State"=w27, "Velocity Count out"=w33, "Detector counter out"=w31, "Timeout count out"=w30, "Measured Charge Out"=w29, "High Correlation Out"=w28, "Plates"=w26, "Offset Out"=w21, "Measured Velocity Out"=w20, "Delay1"=w5, "Out1"=w6, "Final Delay Count Out"=w9) -> (→"Output Cluster":T3)
